vi "BMU诊断标定.vi"(5 "timeout":u32, 6 "Socket":dbl, 7 "通用配置?":bool, 8 "CAN端口":u16(ring), 9 "设备索引号":u16(ring), 10 "CAN卡类型":u32(ring)=21, 11 "从板号":u8=1) -> (3 "成功?":bool)   [LabVIEW 2013] (continued)
              tunnel: [T21."从板信息" ("等级 2") T21."从板信息" ("等级 2") T21."从板信息" ("等级 2") T21."从板信息" ("等级 2") T21."从板信息" ("等级 2") T21."从板信息" ("等级 2") T21."从板信息" ("等级 2") T21."一级故障阀值" ("等级 2") T21."二级故障阀值" ("等级 2") T21."三级故障阀值" ("等级 2") T21."快换参数" ("等级 2") T21."快换参数" ("等级 2") T21."快换参数" ("等级 2") T21."快换参数" ("等级 2") T21."快换参数" ("等级 2") T21."快换参数" ("等级 2") T21."快换参数" ("等级 2") T21."快换参数" ("等级 2") T14."均衡参数" ("等级 2") T14."均衡参数" ("等级 2") T14."均衡参数" ("等级 2") T21."从板信息" ("等级 2")] -> w2480
              tunnel: [w2493 w2503 w2517 w2532 w2567 w2604 w2641 w2665 w2678 w2691 w2704 w2730 w2744 w2760 w2777 w2794 w2812 w2831 w2848 w2861 w2875 w2890] -> w2479
              tunnel: [w2485 w2495 w2505 w2519 w2554 w2591 w2628 w2676 w2678 w2691 w2704 w2730 w2744 w2760 w2777 w2794 w2812 w2831 w2848 w2861 w2875 w2889] -> w2478
              tunnel: [w2485 w2495 w2505 w2519 w2554 w2591 w2628 w2665 w2689 w2691 w2704 w2730 w2744 w2760 w2777 w2794 w2812 w2831 w2848 w2861 w2875 w2889] -> w2477
              tunnel: [w2485 w2495 w2505 w2519 w2554 w2591 w2628 w2665 w2678 w2702 w2704 w2730 w2744 w2760 w2777 w2794 w2812 w2831 w2848 w2861 w2875 w2889] -> w2476
              tunnel: [w2485 w2495 w2505 w2519 w2554 w2591 w2628 w2665 w2678 w2691 w2728 w2742 w2758 w2775 w2792 w2810 w2829 w2846 w2848 w2861 w2875 w2889] -> w2475
              tunnel: [w2490 w2496 w2512 w2526 w2561 w2598 w2635 w2672 w2685 w2698 w2713 w2735 w2750 w2764 w2782 w2797 w2817 w2835 w2851 w2865 w2880 w2889] -> w2474
              tunnel: [w2487 w2496 w2511 w2525 w2560 w2597 w2634 w2671 w2684 w2697 w2705 w2734 w2749 w2763 w2783 w2798 w2816 w2834 w2850 w2864 w2879 w2889] -> w2473
              tunnel: w2470 -> [_ w2500 w2508 w2522 w2557 w2594 w2631 w2667 w2681 w2694 w2725 w2738 w2753 w2768 w2786 w2802 w2820 w2839 w2854 w2868 w2882 _]
              tunnel: [w2485 w2495 w2505 w2519 w2554 w2591 w2628 w2665 w2678 w2691 w2704 w2730 w2744 w2760 w2777 w2794 w2812 w2831 w2849 w2862 w2876 w2889] -> w2469
              frame "从板号" {
                w2492 = 2
                w2485 = FALSE ("1 6")
                n1778 = property on="项目信息 2" class="Tbl (严格)"("Disabled"=w2492) -> ()  [unwired: 2 in, 2 out]
                n1779 = property on="加热控制参数" class="Clust (严格)"("Disabled"=w2492) -> ()  [unwired: 2 in, 2 out]
                n1780 = property on="从板号" class="DigNum (严格)"("NumText.BGColor"=u32 6618880) -> ()  [unwired: 2 in, 2 out]
                n1781 = global read "功能码全局.vi" "16"() -> (w2489:bool[])
                n1782 = Index Array(array=w2489, index #1=4 ("索引"), index #2=6 ("索引")) -> (element #1=w2490:bool, element #2=w2487:bool)
                n1783 = Not(x=w2485) -> (.not. x?=w2493:bool)
              }
              frame "从板信息" {
                w2495 = FALSE ("1 6")
                n1784 = Select(t=0, s=w2500, f=1) -> (s? t:f=w2499:i32)
                n1785 = property on="从板号" class="DigNum (严格)"("NumText.BGColor"=u32 16777215) -> ()  [unwired: 2 in, 2 out]
                n1786 = property on="项目信息 2" class="Tbl (严格)"("Disabled"=w2499) -> ()  [unwired: 2 in, 2 out]
                n1787 = property on="加热控制参数" class="Clust (严格)"("Disabled"=w2499) -> ()  [unwired: 2 in, 2 out]
                n1788 = Not(x=w2495) -> (.not. x?=w2503:bool)
                n1789 = local read "从板项目信息"() -> (w2497:bool)
                n1790 = Not(x=w2497) -> (.not. x?=w2496:bool)
              }
              frame "风机关闭温差", "风机关闭温度", "风机开启温差", "风机开启温度", "加热关闭温差", "加热关闭温度", "加热开启温度", "加热控制参数" {
                w2505 = FALSE ("1 6")
                n1791 = property on="从板号" class="DigNum (严格)"("NumText.BGColor"=u32 16777215) -> ()  [unwired: 2 in, 2 out]
                n1792 = Select(t=0, s=w2508, f=1) -> (s? t:f=w2507:i32)
                n1793 = property on="项目信息 2" class="Tbl (严格)"("Disabled"=2) -> ()  [unwired: 2 in, 2 out]
                n1794 = property on="加热控制参数" class="Clust (严格)"("Disabled"=w2507) -> ()  [unwired: 2 in, 2 out]
                n1795 = global read "功能码全局.vi" "16"() -> (w2514:bool[])
                n1796 = Index Array(array=w2514, index #1=5 ("索引"), index #2=7 ("索引")) -> (element #1=w2512:bool, element #2=w2511:bool)
                n1797 = Not(x=w2505) -> (.not. x?=w2517:bool)
              }
              frame "电压个数" {
                w2519 = FALSE ("1 6")
                n1798 = property on="从板号" class="DigNum (严格)"("NumText.BGColor"=u32 16777215) -> ()  [unwired: 2 in, 2 out]
                n1799 = control-ref of="项目信息 2"() -> (w2530:refnum<vi>)
                n1800 = stacked-sequence {
                  tunnel: w2530 -> [w2537 w2539 w2548]
                  frame #0 {
                    n1801 = Bundle(0, 0) -> (w2536:cluster{i32, i32})  [unwired: 1 out]
                    n1802 = property class="Tbl (严格)"(reference=w2537, "Index Values"=w2536) -> ()  [unwired: 1 in, 2 out]
                  }
                  frame #1 {
                    n1803 = for {
                      N: 40 -> [_]
                      tunnel: w2539 -> [w2546]
                      i -> [w2541]
                      n1804 = Compound Arithmetic op=ADD(0 ("值"), w2541) -> (w2543:i32)
                      n1805 = Bundle(w2543, 0) -> (w2545:cluster{i32, i32})  [unwired: 1 out]
                      n1806 = property class="Tbl (严格)"(reference=w2546, "Active Cell"=w2545, "Cell BG Color"=u32 16448250) -> ()  [unwired: 1 in, 2 out]
                    }
                  }
                  frame #2 {
                    n1807 = for {
                      N: 1 -> [_]
                      tunnel: w2548 -> [w2553]
                      i -> [w2549]
                      n1808 = Bundle(w2549, 0) -> (w2552:cluster{i32, i32})  [unwired: 1 out]
                      n1809 = property class="Tbl (严格)"(reference=w2553, "Active Cell"=w2552, "Cell BG Color"=u32 6618880) -> ()  [unwired: 1 in, 2 out]
                    }
                  }
                }
                n1810 = Select(t=0, s=w2522, f=1) -> (s? t:f=w2521:i32)
                n1811 = property on="项目信息 2" class="Tbl (严格)"("Disabled"=w2521) -> ()  [unwired: 2 in, 2 out]
                n1812 = property on="加热控制参数" class="Clust (严格)"("Disabled"=2) -> ()  [unwired: 2 in, 2 out]
                n1813 = global read "功能码全局.vi" "15"() -> (w2528:bool[])
                n1814 = Index Array(array=w2528, index #1=0 ("索引"), index #2=4 ("索引")) -> (element #1=w2526:bool, element #2=w2525:bool)
                n1815 = Not(x=w2519) -> (.not. x?=w2532:bool)
              }
              frame "通道电压节数" {
                w2554 = FALSE ("1 6")
                n1816 = property on="从板号" class="DigNum (严格)"("NumText.BGColor"=u32 16777215) -> ()  [unwired: 2 in, 2 out]
                n1817 = control-ref of="项目信息 2"() -> (w2565:refnum<vi>)
                n1818 = stacked-sequence {
                  tunnel: w2565 -> [w2572 w2574 w2583]
                  frame #0 {
                    n1819 = Bundle(22, 0) -> (w2571:cluster{i32, i32})  [unwired: 1 out]
                    n1820 = property class="Tbl (严格)"(reference=w2572, "Index Values"=w2571) -> ()  [unwired: 1 in, 2 out]
                  }
                  frame #1 {
                    n1821 = for {
                      N: 40 -> [_]
                      tunnel: w2574 -> [w2581]
                      i -> [w2576]
                      n1822 = Compound Arithmetic op=ADD(0 ("值"), w2576) -> (w2578:i32)
                      n1823 = Bundle(w2578, 0) -> (w2580:cluster{i32, i32})  [unwired: 1 out]
                      n1824 = property class="Tbl (严格)"(reference=w2581, "Active Cell"=w2580, "Cell BG Color"=u32 16448250) -> ()  [unwired: 1 in, 2 out]
                    }
                  }
                  frame #2 {
                    n1825 = for {
                      N: 5 -> [_]
                      tunnel: w2583 -> [w2590]
                      i -> [w2586]
                      n1826 = Add(x=22, y=w2586) -> (x+y=w2585:i32)
                      n1827 = Bundle(w2585, 0) -> (w2589:cluster{i32, i32})  [unwired: 1 out]
                      n1828 = property class="Tbl (严格)"(reference=w2590, "Active Cell"=w2589, "Cell BG Color"=u32 6618880) -> ()  [unwired: 1 in, 2 out]
                    }
                  }
                }
                n1829 = Select(t=0, s=w2557, f=1) -> (s? t:f=w2556:i32)
                n1830 = property on="项目信息 2" class="Tbl (严格)"("Disabled"=w2556) -> ()  [unwired: 2 in, 2 out]
                n1831 = property on="加热控制参数" class="Clust (严格)"("Disabled"=2) -> ()  [unwired: 2 in, 2 out]
                n1832 = global read "功能码全局.vi" "15"() -> (w2563:bool[])
                n1833 = Index Array(array=w2563, index #1=1 ("索引"), index #2=5 ("索引")) -> (element #1=w2561:bool, element #2=w2560:bool)
                n1834 = Not(x=w2554) -> (.not. x?=w2567:bool)
              }
              frame "保险位置" {
                w2591 = FALSE ("1 6")
                n1835 = control-ref of="项目信息 2"() -> (w2602:refnum<vi>)
                n1836 = stacked-sequence {
                  tunnel: w2602 -> [w2609 w2611 w2620]
                  frame #0 {
                    n1837 = Bundle(0, 0) -> (w2608:cluster{i32, i32})  [unwired: 1 out]
                    n1838 = property class="Tbl (严格)"(reference=w2609, "Index Values"=w2608) -> ()  [unwired: 1 in, 2 out]
                  }
                  frame #1 {
                    n1839 = for {
                      N: 40 -> [_]
                      tunnel: w2611 -> [w2618]
                      i -> [w2614]
                      n1840 = Add(x=2, y=w2614) -> (x+y=w2613:i32)
                      n1841 = Bundle(w2613, 0) -> (w2617:cluster{i32, i32})  [unwired: 1 out]
                      n1842 = property class="Tbl (严格)"(reference=w2618, "Active Cell"=w2617, "Cell BG Color"=u32 16448250) -> ()  [unwired: 1 in, 2 out]
                    }
                  }
                  frame #2 {
                    n1843 = for {
                      N: 20 -> [_]
                      tunnel: w2620 -> [w2627]
                      i -> [w2623]
                      n1844 = Add(x=2, y=w2623) -> (x+y=w2622:i32)
                      n1845 = Bundle(w2622, 0) -> (w2626:cluster{i32, i32})  [unwired: 1 out]
                      n1846 = property class="Tbl (严格)"(reference=w2627, "Active Cell"=w2626, "Cell BG Color"=u32 6618880) -> ()  [unwired: 1 in, 2 out]
                    }
                  }
                }
                n1847 = property on="从板号" class="DigNum (严格)"("NumText.BGColor"=u32 16777215) -> ()  [unwired: 2 in, 2 out]
                n1848 = Select(t=0, s=w2594, f=1) -> (s? t:f=w2593:i32)
                n1849 = property on="项目信息 2" class="Tbl (严格)"("Disabled"=w2593) -> ()  [unwired: 2 in, 2 out]
                n1850 = property on="加热控制参数" class="Clust (严格)"("Disabled"=2) -> ()  [unwired: 2 in, 2 out]
                n1851 = global read "功能码全局.vi" "15"() -> (w2600:bool[])
                n1852 = Index Array(array=w2600, index #1=2 ("索引"), index #2=6 ("索引")) -> (element #1=w2598:bool, element #2=w2597:bool)
                n1853 = Not(x=w2591) -> (.not. x?=w2604:bool)
              }
              frame "温度个数" {
                w2628 = FALSE ("1 6")
                n1854 = control-ref of="项目信息 2"() -> (w2639:refnum<vi>)
                n1855 = stacked-sequence {
                  tunnel: w2639 -> [w2646 w2647 w2657]
                  frame #0 {
                    n1856 = Bundle(0, 0) -> (w2645:cluster{i32, i32})  [unwired: 1 out]
                    n1857 = property class="Tbl (严格)"(reference=w2646, "Index Values"=w2645) -> ()  [unwired: 1 in, 2 out]
                  }
                  frame #1 {
                    n1858 = for {
                      N: 40 -> [_]
                      tunnel: w2647 -> [w2655]
                      i -> [w2650]
                      n1859 = Compound Arithmetic op=ADD(0 ("值"), w2650) -> (w2652:i32)
                      n1860 = Bundle(w2652, 0) -> (w2654:cluster{i32, i32})  [unwired: 1 out]
                      n1861 = property class="Tbl (严格)"(reference=w2655, "Active Cell"=w2654, "Cell BG Color"=u32 16448250) -> ()  [unwired: 1 in, 2 out]
                    }
                  }
                  frame #2 {
                    n1862 = for {
                      N: 1 -> [_]
                      tunnel: w2657 -> [w2664]
                      i -> [w2660]
                      n1863 = Add(x=1, y=w2660) -> (x+y=w2659:i32)
                      n1864 = Bundle(w2659, 0) -> (w2663:cluster{i32, i32})  [unwired: 1 out]
                      n1865 = property class="Tbl (严格)"(reference=w2664, "Active Cell"=w2663, "Cell BG Color"=u32 6618880) -> ()  [unwired: 1 in, 2 out]
                    }
                  }
                }
                n1866 = Select(t=0, s=w2631, f=1) -> (s? t:f=w2630:i32)
                n1867 = property on="项目信息 2" class="Tbl (严格)"("Disabled"=w2630) -> ()  [unwired: 2 in, 2 out]
                n1868 = property on="加热控制参数" class="Clust (严格)"("Disabled"=2) -> ()  [unwired: 2 in, 2 out]
                n1869 = property on="从板号" class="DigNum (严格)"("NumText.BGColor"=u32 16777215) -> ()  [unwired: 2 in, 2 out]
                n1870 = global read "功能码全局.vi" "15"() -> (w2637:bool[])
                n1871 = Index Array(array=w2637, index #1=3 ("索引"), index #2=7 ("索引")) -> (element #1=w2635:bool, element #2=w2634:bool)
                n1872 = Not(x=w2628) -> (.not. x?=w2641:bool)
              }
              frame "SOC过低", "电压不均衡", "电压过低", "电压过高", "温度不均衡", "温度过低", "温度过高", "一级故障阀值" {
                w2665 = FALSE ("1 6")
                n1873 = property on="从板号" class="DigNum (严格)"("NumText.BGColor"=u32 16777215) -> ()  [unwired: 2 in, 2 out]
                n1874 = Select(t=0, s=w2667, f=1) -> (s? t:f=w2668:i32)
                n1875 = property on="一级故障 6" class="Clust (严格)"("DisabledEnum"=w2668) -> ()  [unwired: 2 in, 2 out]
                n1876 = global read "功能码全局.vi" "18"() -> (w2674:bool[])
                n1877 = Index Array(array=w2674, index #1=2 ("索引"), index #2=5 ("索引")) -> (element #1=w2672:bool, element #2=w2671:bool)
                n1878 = Not(x=w2665) -> (.not. x?=w2676:bool)
              }
              frame "SOC过低(2)", "电压不均衡(2)", "电压过低(2)", "电压过高(2)", "二级故障阀值", "温度不均衡(2)", "温度过低(2)", "温度过高(2)" {
                w2678 = FALSE ("1 6")
                n1879 = property on="从板号" class="DigNum (严格)"("NumText.BGColor"=u32 16777215) -> ()  [unwired: 2 in, 2 out]
                n1880 = Select(t=0, s=w2681, f=1) -> (s? t:f=w2680:i32)
                n1881 = property on="一级故障 7" class="Clust (严格)"("DisabledEnum"=w2680) -> ()  [unwired: 2 in, 2 out]
                n1882 = global read "功能码全局.vi" "18"() -> (w2687:bool[])
                n1883 = Index Array(array=w2687, index #1=3 ("索引"), index #2=6 ("索引")) -> (element #1=w2685:bool, element #2=w2684:bool)
                n1884 = Not(x=w2678) -> (.not. x?=w2689:bool)
              }
              frame "SOC过低(3)", "电压不均衡(3)", "电压过低(3)", "电压过高(3)", "三级故障阀值", "温度不均衡(3)", "温度过低(3)", "温度过高(3)" {
                w2691 = FALSE ("1 6")
                n1885 = property on="从板号" class="DigNum (严格)"("NumText.BGColor"=u32 16777215) -> ()  [unwired: 2 in, 2 out]
                n1886 = Select(t=0, s=w2694, f=1) -> (s? t:f=w2693:i32)
                n1887 = property on="一级故障 8" class="Clust (严格)"("DisabledEnum"=w2693) -> ()  [unwired: 2 in, 2 out]
                n1888 = global read "功能码全局.vi" "18"() -> (w2700:bool[])
                n1889 = Index Array(array=w2700, index #1=4 ("索引"), index #2=7 ("索引")) -> (element #1=w2698:bool, element #2=w2697:bool)
                n1890 = Not(x=w2691) -> (.not. x?=w2702:bool)
              }
              frame "快换参数" {
                w2704 = FALSE ("1 6")
                n1891 = Select(t=0, s=w2725, f=1) -> (s? t:f=w2724:i32)
                n1892 = property on="电池组信息" class="Clust (严格)"("Disabled"=w2724) -> ()  [unwired: 2 in, 2 out]
                n1893 = property on="从板号" class="DigNum (严格)"("NumText.BGColor"=u32 16777215) -> ()  [unwired: 2 in, 2 out]
                n1894 = global read "功能码全局.vi" "24"() -> (w2721:bool[])
                n1895 = global read "功能码全局.vi" "23"() -> (w2722:bool[])
                n1896 = Index Array(array=w2721) -> (element #3=w2711:bool, element #4=w2710:bool, element #5=w2709:bool, element #6=w2708:bool, element #7=w2707:bool, element #8=w2706:bool)  [unwired: 8 in, 2 out]
                n1897 = Index Array(array=w2722) -> (element #3=w2720:bool, element #4=w2719:bool, element #5=w2718:bool, element #6=w2717:bool, element #7=w2716:bool, element #8=w2715:bool)  [unwired: 8 in, 2 out]
                n1898 = Build Array(w2711, w2710, w2709, w2708, w2707, w2706) -> (w2712:bool[])
                n1899 = Build Array(w2720, w2719, w2718, w2717, w2716, w2715) -> (w2714:bool[])
                n1900 = And Array Elements(Boolean array=w2712) -> (logical AND=w2705:bool)
                n1901 = And Array Elements(Boolean array=w2714) -> (logical AND=w2713:bool)
                n1902 = Not(x=w2704) -> (.not. x?=w2728:bool)
              }
              frame "电池包信息1" {
                w2733 = 2
                w2741 = 2
                w2732 = 2
                w2730 = FALSE ("1 6")
                n1903 = Select(t=0, s=w2738, f=1) -> (s? t:f=w2731:i32)
                n1904 = property on="串联数" class="DigNum (严格)"("Disabled"=w2731) -> ()  [unwired: 2 in, 2 out]
                n1905 = property on="并联数" class="DigNum (严格)"("Disabled"=w2731) -> ()  [unwired: 2 in, 2 out]
                n1906 = property on="电池厂家" class="DigNum (严格)"("Disabled"=w2731) -> ()  [unwired: 2 in, 2 out]
                n1907 = property on="电池类型" class="DigNum (严格)"("Disabled"=w2731) -> ()  [unwired: 2 in, 2 out]
                n1908 = property on="额定能量" class="DigNum (严格)"("Disabled"=w2731) -> ()  [unwired: 2 in, 2 out]
                n1909 = property on="额定容量" class="DigNum (严格)"("Disabled"=w2731) -> ()  [unwired: 2 in, 2 out]
                n1910 = property on="实际容量" class="DigNum (严格)"("Disabled"=w2731) -> ()  [unwired: 2 in, 2 out]
                n1911 = property on="电池组信息" class="Clust (严格)"("Disabled"=w2731) -> ()  [unwired: 2 in, 2 out]
                n1912 = property on="生产日期" class="Str"("DisabledEnum"=w2731) -> ()  [unwired: 2 in, 2 out]
                n1913 = property on="车牌号" class="Str"("DisabledEnum"=w2732) -> ()  [unwired: 2 in, 2 out]
                n1914 = property on="产权标识" class="DigNum (严格)"("Disabled"=w2731) -> ()  [unwired: 2 in, 2 out]
                n1915 = property on="应用车型" class="DigNum (严格)"("Disabled"=w2731) -> ()  [unwired: 2 in, 2 out]
                n1916 = property on="额定总压" class="DigNum (严格)"("Disabled"=w2731) -> ()  [unwired: 2 in, 2 out]
                n1917 = property on="电池包序号" class="DigNum (严格)"("DisabledEnum"=w2731) -> ()  [unwired: 2 in, 2 out]
                n1918 = property on="电池包组号" class="DigNum (严格)"("DisabledEnum"=w2732) -> ()  [unwired: 2 in, 2 out]
                n1919 = property on="最大允许单体电压" class="DigNum (严格)"("Disabled"=w2741) -> ()  [unwired: 2 in, 2 out]
                n1920 = property on="最大允许总电压" class="DigNum (严格)"("Disabled"=w2741) -> ()  [unwired: 2 in, 2 out]
                n1921 = property on="最大允许温度" class="DigNum (严格)"("Disabled"=w2741) -> ()  [unwired: 2 in, 2 out]
                n1922 = property on="最小允许温度" class="DigNum (严格)"("Disabled"=w2741) -> ()  [unwired: 2 in, 2 out]
                n1923 = property on="最大允许充电电流" class="DigNum (严格)"("Disabled"=w2741) -> ()  [unwired: 2 in, 2 out]
                n1924 = property on="最小允许充电电流" class="DigNum (严格)"("Disabled"=w2741) -> ()  [unwired: 2 in, 2 out]
                n1925 = property on="最小允许单体电压" class="DigNum (严格)"("Disabled"=w2741) -> ()  [unwired: 2 in, 2 out]
                n1926 = property on="电流步长" class="DigNum (严格)"("Disabled"=w2741) -> ()  [unwired: 2 in, 2 out]
                n1927 = property on="SOC" class="DigNum (严格)"("Disabled"=w2741) -> ()  [unwired: 2 in, 2 out]
                n1928 = property on="充电总安时" class="DigNum (严格)"("Disabled"=w2741) -> ()  [unwired: 2 in, 2 out]
                n1929 = property on="放电总安时" class="DigNum (严格)"("Disabled"=w2741) -> ()  [unwired: 2 in, 2 out]
                n1930 = property on="放空次数" class="DigNum (严格)"("DisabledEnum"=w2733) -> ()  [unwired: 2 in, 2 out]
                n1931 = property on="充满次数" class="DigNum (严格)"("DisabledEnum"=w2733) -> ()  [unwired: 2 in, 2 out]
                n1932 = property on="充电次数" class="DigNum (严格)"("DisabledEnum"=w2733) -> ()  [unwired: 2 in, 2 out]
                n1933 = global read "功能码全局.vi" "24"() -> (w2736:bool[])
                n1934 = global read "功能码全局.vi" "23"() -> (w2737:bool[])
                n1935 = Index Array(array=w2736) -> (element #3=w2734:bool)  [unwired: 8 in, 7 out]
                n1936 = Index Array(array=w2737) -> (element #3=w2735:bool)  [unwired: 8 in, 7 out]
                n1937 = Not(x=w2730) -> (.not. x?=w2742:bool)
              }
              frame "电池包组号" {
                w2747 = 2
                w2746 = 2
                w2756 = 2
                w2748 = 2
                w2757 = 2
                w2744 = FALSE ("1 6")
                n1938 = property on="串联数" class="DigNum (严格)"("Disabled"=w2757) -> ()  [unwired: 2 in, 2 out]
                n1939 = property on="并联数" class="DigNum (严格)"("Disabled"=w2757) -> ()  [unwired: 2 in, 2 out]
                n1940 = property on="电池厂家" class="DigNum (严格)"("Disabled"=w2757) -> ()  [unwired: 2 in, 2 out]
                n1941 = property on="电池类型" class="DigNum (严格)"("Disabled"=w2757) -> ()  [unwired: 2 in, 2 out]
                n1942 = property on="额定能量" class="DigNum (严格)"("Disabled"=w2757) -> ()  [unwired: 2 in, 2 out]
                n1943 = property on="额定容量" class="DigNum (严格)"("Disabled"=w2757) -> ()  [unwired: 2 in, 2 out]
                n1944 = property on="实际容量" class="DigNum (严格)"("Disabled"=w2757) -> ()  [unwired: 2 in, 2 out]
                n1945 = Select(t=0, s=w2753, f=1) -> (s? t:f=w2745:i32)
                n1946 = property on="生产日期" class="Str"("DisabledEnum"=w2747) -> ()  [unwired: 2 in, 2 out]
                n1947 = property on="电池包序号" class="DigNum (严格)"("DisabledEnum"=w2747) -> ()  [unwired: 2 in, 2 out]
                n1948 = property on="车牌号" class="Str"("DisabledEnum"=w2747) -> ()  [unwired: 2 in, 2 out]
                n1949 = property on="电池包组号" class="DigNum (严格)"("DisabledEnum"=w2745) -> ()  [unwired: 2 in, 2 out]
                n1950 = property on="电池组信息" class="Clust (严格)"("Disabled"=w2745) -> ()  [unwired: 2 in, 2 out]
                n1951 = property on="产权标识" class="DigNum (严格)"("Disabled"=w2748) -> ()  [unwired: 2 in, 2 out]
                n1952 = property on="应用车型" class="DigNum (严格)"("Disabled"=w2748) -> ()  [unwired: 2 in, 2 out]
                n1953 = property on="额定总压" class="DigNum (严格)"("Disabled"=w2748) -> ()  [unwired: 2 in, 2 out]
                n1954 = property on="放空次数" class="DigNum (严格)"("DisabledEnum"=w2746) -> ()  [unwired: 2 in, 2 out]
                n1955 = property on="充满次数" class="DigNum (严格)"("DisabledEnum"=w2746) -> ()  [unwired: 2 in, 2 out]
                n1956 = property on="充电次数" class="DigNum (严格)"("DisabledEnum"=w2746) -> ()  [unwired: 2 in, 2 out]
                n1957 = property on="最大允许单体电压" class="DigNum (严格)"("Disabled"=w2756) -> ()  [unwired: 2 in, 2 out]
                n1958 = property on="最大允许总电压" class="DigNum (严格)"("Disabled"=w2756) -> ()  [unwired: 2 in, 2 out]
                n1959 = property on="最大允许温度" class="DigNum (严格)"("Disabled"=w2756) -> ()  [unwired: 2 in, 2 out]
                n1960 = property on="最小允许温度" class="DigNum (严格)"("Disabled"=w2756) -> ()  [unwired: 2 in, 2 out]
                n1961 = property on="最大允许充电电流" class="DigNum (严格)"("Disabled"=w2756) -> ()  [unwired: 2 in, 2 out]
                n1962 = property on="最小允许充电电流" class="DigNum (严格)"("Disabled"=w2756) -> ()  [unwired: 2 in, 2 out]
                n1963 = property on="最小允许单体电压" class="DigNum (严格)"("Disabled"=w2756) -> ()  [unwired: 2 in, 2 out]
                n1964 = property on="电流步长" class="DigNum (严格)"("Disabled"=w2756) -> ()  [unwired: 2 in, 2 out]
                n1965 = property on="SOC" class="DigNum (严格)"("Disabled"=w2756) -> ()  [unwired: 2 in, 2 out]
                n1966 = property on="充电总安时" class="DigNum (严格)"("Disabled"=w2756) -> ()  [unwired: 2 in, 2 out]
                n1967 = property on="放电总安时" class="DigNum (严格)"("Disabled"=w2756) -> ()  [unwired: 2 in, 2 out]
                n1968 = global read "功能码全局.vi" "24"() -> (w2751:bool[])
                n1969 = global read "功能码全局.vi" "23"() -> (w2752:bool[])
                n1970 = Index Array(array=w2751) -> (element #3=w2749:bool)  [unwired: 8 in, 7 out]
                n1971 = Index Array(array=w2752) -> (element #3=w2750:bool)  [unwired: 8 in, 7 out]
                n1972 = Not(x=w2744) -> (.not. x?=w2758:bool)
              }
              frame "充放电安时" {
                w2762 = 2
                w2761 = 2
                w2771 = 2
                w2772 = 2
                w2774 = 2
                w2760 = FALSE ("1 6")
                n1973 = property on="串联数" class="DigNum (严格)"("Disabled"=w2774) -> ()  [unwired: 2 in, 2 out]
                n1974 = property on="并联数" class="DigNum (严格)"("Disabled"=w2774) -> ()  [unwired: 2 in, 2 out]
                n1975 = property on="电池厂家" class="DigNum (严格)"("Disabled"=w2774) -> ()  [unwired: 2 in, 2 out]
                n1976 = property on="电池类型" class="DigNum (严格)"("Disabled"=w2774) -> ()  [unwired: 2 in, 2 out]
                n1977 = property on="额定能量" class="DigNum (严格)"("Disabled"=w2774) -> ()  [unwired: 2 in, 2 out]
                n1978 = property on="额定容量" class="DigNum (严格)"("Disabled"=w2774) -> ()  [unwired: 2 in, 2 out]
                n1979 = property on="实际容量" class="DigNum (严格)"("Disabled"=w2774) -> ()  [unwired: 2 in, 2 out]
                n1980 = Select(t=0, s=w2768, f=1) -> (s? t:f=w2767:i32)
                n1981 = property on="生产日期" class="Str"("DisabledEnum"=w2762) -> ()  [unwired: 2 in, 2 out]
                n1982 = property on="电池包序号" class="DigNum (严格)"("DisabledEnum"=w2762) -> ()  [unwired: 2 in, 2 out]
                n1983 = property on="车牌号" class="Str"("DisabledEnum"=w2762) -> ()  [unwired: 2 in, 2 out]
                n1984 = property on="电池包组号" class="DigNum (严格)"("DisabledEnum"=w2762) -> ()  [unwired: 2 in, 2 out]
                n1985 = property on="电池组信息" class="Clust (严格)"("Disabled"=w2767) -> ()  [unwired: 2 in, 2 out]
                n1986 = property on="额定总压" class="DigNum (严格)"("Disabled"=2) -> ()  [unwired: 2 in, 2 out]
                n1987 = property on="产权标识" class="DigNum (严格)"("Disabled"=w2772) -> ()  [unwired: 2 in, 2 out]
                n1988 = property on="应用车型" class="DigNum (严格)"("Disabled"=w2772) -> ()  [unwired: 2 in, 2 out]
                n1989 = property on="放空次数" class="DigNum (严格)"("DisabledEnum"=w2761) -> ()  [unwired: 2 in, 2 out]
                n1990 = property on="充满次数" class="DigNum (严格)"("DisabledEnum"=w2761) -> ()  [unwired: 2 in, 2 out]
                n1991 = property on="充电次数" class="DigNum (严格)"("DisabledEnum"=w2761) -> ()  [unwired: 2 in, 2 out]
                n1992 = property on="最大允许单体电压" class="DigNum (严格)"("Disabled"=w2771) -> ()  [unwired: 2 in, 2 out]
                n1993 = property on="最大允许总电压" class="DigNum (严格)"("Disabled"=w2771) -> ()  [unwired: 2 in, 2 out]
                n1994 = property on="最大允许温度" class="DigNum (严格)"("Disabled"=w2771) -> ()  [unwired: 2 in, 2 out]
                n1995 = property on="最小允许温度" class="DigNum (严格)"("Disabled"=w2771) -> ()  [unwired: 2 in, 2 out]
                n1996 = property on="最大允许充电电流" class="DigNum (严格)"("Disabled"=w2771) -> ()  [unwired: 2 in, 2 out]
                n1997 = property on="最小允许充电电流" class="DigNum (严格)"("Disabled"=w2771) -> ()  [unwired: 2 in, 2 out]
                n1998 = property on="最小允许单体电压" class="DigNum (严格)"("Disabled"=w2771) -> ()  [unwired: 2 in, 2 out]
                n1999 = property on="电流步长" class="DigNum (严格)"("Disabled"=w2771) -> ()  [unwired: 2 in, 2 out]
                n2000 = property on="SOC" class="DigNum (严格)"("Disabled"=w2771) -> ()  [unwired: 2 in, 2 out]
                n2001 = property on="充电总安时" class="DigNum (严格)"("Disabled"=w2767) -> ()  [unwired: 2 in, 2 out]
                n2002 = property on="放电总安时" class="DigNum (严格)"("Disabled"=w2767) -> ()  [unwired: 2 in, 2 out]
                n2003 = Not(x=w2760) -> (.not. x?=w2775:bool)
                n2004 = global read "功能码全局.vi" "24"() -> (w2765:bool[])
                n2005 = global read "功能码全局.vi" "23"() -> (w2766:bool[])
                n2006 = Index Array(array=w2765) -> (element #7=w2763:bool)  [unwired: 8 in, 7 out]
                n2007 = Index Array(array=w2766) -> (element #7=w2764:bool)  [unwired: 8 in, 7 out]
              }
              frame "充电次数" {
                w2780 = 2
                w2789 = 2
                w2790 = 2
                w2781 = 2
                w2791 = 2
                w2777 = FALSE ("1 6")
                n2008 = property on="串联数" class="DigNum (严格)"("Disabled"=w2791) -> ()  [unwired: 2 in, 2 out]
                n2009 = property on="并联数" class="DigNum (严格)"("Disabled"=w2791) -> ()  [unwired: 2 in, 2 out]
                n2010 = property on="电池厂家" class="DigNum (严格)"("Disabled"=w2791) -> ()  [unwired: 2 in, 2 out]
                n2011 = property on="电池类型" class="DigNum (严格)"("Disabled"=w2791) -> ()  [unwired: 2 in, 2 out]
                n2012 = property on="额定能量" class="DigNum (严格)"("Disabled"=w2791) -> ()  [unwired: 2 in, 2 out]
                n2013 = property on="额定容量" class="DigNum (严格)"("Disabled"=w2791) -> ()  [unwired: 2 in, 2 out]
                n2014 = property on="实际容量" class="DigNum (严格)"("Disabled"=w2791) -> ()  [unwired: 2 in, 2 out]
                n2015 = Select(t=0, s=w2786, f=1) -> (s? t:f=w2778:i32)
                n2016 = property on="生产日期" class="Str"("DisabledEnum"=w2780) -> ()  [unwired: 2 in, 2 out]
                n2017 = property on="电池包序号" class="DigNum (严格)"("DisabledEnum"=w2780) -> ()  [unwired: 2 in, 2 out]
                n2018 = property on="车牌号" class="Str"("DisabledEnum"=w2780) -> ()  [unwired: 2 in, 2 out]
                n2019 = property on="电池组信息" class="Clust (严格)"("Disabled"=w2778) -> ()  [unwired: 2 in, 2 out]
                n2020 = property on="电池包组号" class="DigNum (严格)"("DisabledEnum"=w2780) -> ()  [unwired: 2 in, 2 out]
                n2021 = property on="额定总压" class="DigNum (严格)"("Disabled"=w2781) -> ()  [unwired: 2 in, 2 out]
                n2022 = property on="产权标识" class="DigNum (严格)"("Disabled"=w2781) -> ()  [unwired: 2 in, 2 out]
                n2023 = property on="应用车型" class="DigNum (严格)"("Disabled"=w2781) -> ()  [unwired: 2 in, 2 out]
                n2024 = property on="放空次数" class="DigNum (严格)"("DisabledEnum"=w2778) -> (error out=w2779:errorcluster)  [unwired: 2 in, 1 out]
                n2025 = property on="充满次数" class="DigNum (严格)"("DisabledEnum"=w2778) -> ()  [unwired: 2 in, 2 out]
                n2026 = property on="充电次数" class="DigNum (严格)"("DisabledEnum"=w2778) -> ()  [unwired: 2 in, 2 out]
                n2027 = property on="最大允许单体电压" class="DigNum (严格)"("Disabled"=w2790) -> ()  [unwired: 2 in, 2 out]
                n2028 = property on="最大允许总电压" class="DigNum (严格)"("Disabled"=w2790) -> ()  [unwired: 2 in, 2 out]
                n2029 = property on="最大允许温度" class="DigNum (严格)"("Disabled"=w2790) -> ()  [unwired: 2 in, 2 out]
                n2030 = property on="最小允许温度" class="DigNum (严格)"("Disabled"=w2790) -> ()  [unwired: 2 in, 2 out]
                n2031 = property on="最大允许充电电流" class="DigNum (严格)"("Disabled"=w2790) -> ()  [unwired: 2 in, 2 out]
                n2032 = property on="最小允许充电电流" class="DigNum (严格)"(error in=w2779, "Disabled"=w2790) -> ()  [unwired: 1 in, 2 out]
                n2033 = property on="最小允许单体电压" class="DigNum (严格)"("Disabled"=w2790) -> ()  [unwired: 2 in, 2 out]
                n2034 = property on="电流步长" class="DigNum (严格)"("Disabled"=w2790) -> ()  [unwired: 2 in, 2 out]
                n2035 = property on="SOC" class="DigNum (严格)"("Disabled"=w2790) -> ()  [unwired: 2 in, 2 out]
                n2036 = property on="充电总安时" class="DigNum (严格)"("Disabled"=w2789) -> ()  [unwired: 2 in, 2 out]
                n2037 = property on="放电总安时" class="DigNum (严格)"("Disabled"=w2789) -> ()  [unwired: 2 in, 2 out]
                n2038 = Not(x=w2777) -> (.not. x?=w2792:bool)
                n2039 = global read "功能码全局.vi" "24"() -> (w2784:bool[])
                n2040 = global read "功能码全局.vi" "23"() -> (w2785:bool[])
                n2041 = Index Array(array=w2784) -> (element #8=w2783:bool)  [unwired: 8 in, 7 out]
                n2042 = Index Array(array=w2785) -> (element #8=w2782:bool)  [unwired: 8 in, 7 out]
              }
              frame "SOC" {
                w2796 = 2
                w2795 = 2
                w2805 = 2
                w2806 = 2
                w2807 = 2
                w2809 = 2
                w2794 = FALSE ("1 6")
                n2043 = property on="串联数" class="DigNum (严格)"("Disabled"=w2809) -> ()  [unwired: 2 in, 2 out]
                n2044 = property on="并联数" class="DigNum (严格)"("Disabled"=w2809) -> ()  [unwired: 2 in, 2 out]
                n2045 = property on="电池厂家" class="DigNum (严格)"("Disabled"=w2809) -> ()  [unwired: 2 in, 2 out]
                n2046 = property on="电池类型" class="DigNum (严格)"("Disabled"=w2809) -> ()  [unwired: 2 in, 2 out]
                n2047 = property on="额定能量" class="DigNum (严格)"("Disabled"=w2809) -> ()  [unwired: 2 in, 2 out]
                n2048 = property on="额定容量" class="DigNum (严格)"("Disabled"=w2809) -> ()  [unwired: 2 in, 2 out]
                n2049 = property on="实际容量" class="DigNum (严格)"("Disabled"=w2809) -> ()  [unwired: 2 in, 2 out]
                n2050 = Select(t=0, s=w2802, f=1) -> (s? t:f=w2801:i32)
                n2051 = property on="生产日期" class="Str"("DisabledEnum"=w2796) -> ()  [unwired: 2 in, 2 out]
                n2052 = property on="电池包序号" class="DigNum (严格)"("DisabledEnum"=w2796) -> ()  [unwired: 2 in, 2 out]
                n2053 = property on="车牌号" class="Str"("DisabledEnum"=w2796) -> ()  [unwired: 2 in, 2 out]
                n2054 = property on="电池包组号" class="DigNum (严格)"("DisabledEnum"=w2796) -> ()  [unwired: 2 in, 2 out]
                n2055 = property on="电池组信息" class="Clust (严格)"("Disabled"=w2801) -> ()  [unwired: 2 in, 2 out]
                n2056 = property on="SOC" class="DigNum (严格)"("Disabled"=w2801) -> ()  [unwired: 2 in, 2 out]
                n2057 = property on="额定总压" class="DigNum (严格)"("Disabled"=2) -> ()  [unwired: 2 in, 2 out]
                n2058 = property on="产权标识" class="DigNum (严格)"("Disabled"=w2807) -> ()  [unwired: 2 in, 2 out]
                n2059 = property on="应用车型" class="DigNum (严格)"("Disabled"=w2807) -> ()  [unwired: 2 in, 2 out]
                n2060 = property on="放空次数" class="DigNum (严格)"("DisabledEnum"=w2795) -> ()  [unwired: 2 in, 2 out]
                n2061 = property on="充满次数" class="DigNum (严格)"("DisabledEnum"=w2795) -> ()  [unwired: 2 in, 2 out]
                n2062 = property on="充电次数" class="DigNum (严格)"("DisabledEnum"=w2795) -> ()  [unwired: 2 in, 2 out]
                n2063 = property on="最大允许单体电压" class="DigNum (严格)"("Disabled"=w2806) -> ()  [unwired: 2 in, 2 out]
                n2064 = property on="最大允许总电压" class="DigNum (严格)"("Disabled"=w2806) -> ()  [unwired: 2 in, 2 out]
                n2065 = property on="最大允许温度" class="DigNum (严格)"("Disabled"=w2806) -> ()  [unwired: 2 in, 2 out]
                n2066 = property on="最小允许温度" class="DigNum (严格)"("Disabled"=w2806) -> ()  [unwired: 2 in, 2 out]
                n2067 = property on="最大允许充电电流" class="DigNum (严格)"("Disabled"=w2806) -> ()  [unwired: 2 in, 2 out]
                n2068 = property on="最小允许充电电流" class="DigNum (严格)"("Disabled"=w2806) -> ()  [unwired: 2 in, 2 out]
                n2069 = property on="最小允许单体电压" class="DigNum (严格)"("Disabled"=w2806) -> ()  [unwired: 2 in, 2 out]
                n2070 = property on="电流步长" class="DigNum (严格)"("Disabled"=w2806) -> ()  [unwired: 2 in, 2 out]
                n2071 = property on="充电总安时" class="DigNum (严格)"("Disabled"=w2805) -> ()  [unwired: 2 in, 2 out]
                n2072 = property on="放电总安时" class="DigNum (严格)"("Disabled"=w2805) -> ()  [unwired: 2 in, 2 out]
                n2073 = Not(x=w2794) -> (.not. x?=w2810:bool)
                n2074 = global read "功能码全局.vi" "24"() -> (w2799:bool[])
                n2075 = global read "功能码全局.vi" "23"() -> (w2800:bool[])
                n2076 = Index Array(array=w2799) -> (element #6=w2798:bool)  [unwired: 8 in, 7 out]
                n2077 = Index Array(array=w2800) -> (element #6=w2797:bool)  [unwired: 8 in, 7 out]
              }
              frame "车牌号" {
                w2815 = 2
                w2814 = 2
                w2824 = 2
                w2825 = 2
                w2826 = 2
                w2828 = 2
                w2812 = FALSE ("1 6")
                n2078 = property on="串联数" class="DigNum (严格)"("Disabled"=w2828) -> ()  [unwired: 2 in, 2 out]
                n2079 = property on="并联数" class="DigNum (严格)"("Disabled"=w2828) -> ()  [unwired: 2 in, 2 out]
                n2080 = property on="电池厂家" class="DigNum (严格)"("Disabled"=w2828) -> ()  [unwired: 2 in, 2 out]
                n2081 = property on="电池类型" class="DigNum (严格)"("Disabled"=w2828) -> ()  [unwired: 2 in, 2 out]
                n2082 = property on="额定能量" class="DigNum (严格)"("Disabled"=w2828) -> ()  [unwired: 2 in, 2 out]
                n2083 = property on="额定容量" class="DigNum (严格)"("Disabled"=w2828) -> ()  [unwired: 2 in, 2 out]
                n2084 = property on="实际容量" class="DigNum (严格)"("Disabled"=w2828) -> ()  [unwired: 2 in, 2 out]
                n2085 = Select(t=0, s=w2820, f=1) -> (s? t:f=w2813:i32)
                n2086 = property on="生产日期" class="Str"("DisabledEnum"=w2815) -> ()  [unwired: 2 in, 2 out]
                n2087 = property on="电池包序号" class="DigNum (严格)"("DisabledEnum"=w2815) -> ()  [unwired: 2 in, 2 out]
                n2088 = property on="电池包组号" class="DigNum (严格)"("DisabledEnum"=w2815) -> ()  [unwired: 2 in, 2 out]
                n2089 = property on="电池组信息" class="Clust (严格)"("Disabled"=w2813) -> ()  [unwired: 2 in, 2 out]
                n2090 = property on="车牌号" class="Str"("DisabledEnum"=w2813) -> ()  [unwired: 2 in, 2 out]
                n2091 = property on="额定总压" class="DigNum (严格)"("Disabled"=2) -> ()  [unwired: 2 in, 2 out]
                n2092 = property on="产权标识" class="DigNum (严格)"("Disabled"=w2826) -> ()  [unwired: 2 in, 2 out]
                n2093 = property on="应用车型" class="DigNum (严格)"("Disabled"=w2826) -> ()  [unwired: 2 in, 2 out]
                n2094 = property on="放空次数" class="DigNum (严格)"("DisabledEnum"=w2814) -> ()  [unwired: 2 in, 2 out]
                n2095 = property on="充满次数" class="DigNum (严格)"("DisabledEnum"=w2814) -> ()  [unwired: 2 in, 2 out]
                n2096 = property on="充电次数" class="DigNum (严格)"("DisabledEnum"=w2814) -> ()  [unwired: 2 in, 2 out]
                n2097 = property on="最大允许单体电压" class="DigNum (严格)"("Disabled"=w2825) -> ()  [unwired: 2 in, 2 out]
                n2098 = property on="最大允许总电压" class="DigNum (严格)"("Disabled"=w2825) -> ()  [unwired: 2 in, 2 out]
                n2099 = property on="最大允许温度" class="DigNum (严格)"("Disabled"=w2825) -> ()  [unwired: 2 in, 2 out]
                n2100 = property on="最小允许温度" class="DigNum (严格)"("Disabled"=w2825) -> ()  [unwired: 2 in, 2 out]
                n2101 = property on="最大允许充电电流" class="DigNum (严格)"("Disabled"=w2825) -> ()  [unwired: 2 in, 2 out]
                n2102 = property on="最小允许充电电流" class="DigNum (严格)"("Disabled"=w2825) -> ()  [unwired: 2 in, 2 out]
                n2103 = property on="最小允许单体电压" class="DigNum (严格)"("Disabled"=w2825) -> ()  [unwired: 2 in, 2 out]
                n2104 = property on="电流步长" class="DigNum (严格)"("Disabled"=w2825) -> ()  [unwired: 2 in, 2 out]
                n2105 = property on="SOC" class="DigNum (严格)"("Disabled"=2) -> ()  [unwired: 2 in, 2 out]
                n2106 = property on="充电总安时" class="DigNum (严格)"("Disabled"=w2824) -> ()  [unwired: 2 in, 2 out]
                n2107 = property on="放电总安时" class="DigNum (严格)"("Disabled"=w2824) -> ()  [unwired: 2 in, 2 out]
                n2108 = Not(x=w2812) -> (.not. x?=w2829:bool)
                n2109 = global read "功能码全局.vi" "24"() -> (w2818:bool[])
                n2110 = global read "功能码全局.vi" "23"() -> (w2819:bool[])
                n2111 = Index Array(array=w2818) -> (element #5=w2816:bool)  [unwired: 8 in, 7 out]
                n2112 = Index Array(array=w2819) -> (element #5=w2817:bool)  [unwired: 8 in, 7 out]
              }
              frame "充电参数" {
                w2833 = 2
                w2832 = 2
                w2842 = 2
                w2843 = 2
                w2845 = 2
                w2831 = FALSE ("1 6")
                n2113 = property on="串联数" class="DigNum (严格)"("Disabled"=w2845) -> ()  [unwired: 2 in, 2 out]
                n2114 = property on="并联数" class="DigNum (严格)"("Disabled"=w2845) -> ()  [unwired: 2 in, 2 out]
                n2115 = property on="电池厂家" class="DigNum (严格)"("Disabled"=w2845) -> ()  [unwired: 2 in, 2 out]
                n2116 = property on="电池类型" class="DigNum (严格)"("Disabled"=w2845) -> ()  [unwired: 2 in, 2 out]
                n2117 = property on="额定能量" class="DigNum (严格)"("Disabled"=w2845) -> ()  [unwired: 2 in, 2 out]
                n2118 = property on="额定容量" class="DigNum (严格)"("Disabled"=w2845) -> ()  [unwired: 2 in, 2 out]
                n2119 = property on="实际容量" class="DigNum (严格)"("Disabled"=w2845) -> ()  [unwired: 2 in, 2 out]
                n2120 = Select(t=0, s=w2839, f=1) -> (s? t:f=w2838:i32)
                n2121 = property on="生产日期" class="Str"("DisabledEnum"=w2833) -> ()  [unwired: 2 in, 2 out]
                n2122 = property on="电池包序号" class="DigNum (严格)"("DisabledEnum"=w2833) -> ()  [unwired: 2 in, 2 out]
                n2123 = property on="车牌号" class="Str"("DisabledEnum"=w2833) -> ()  [unwired: 2 in, 2 out]
                n2124 = property on="电池组信息" class="Clust (严格)"("Disabled"=w2838) -> ()  [unwired: 2 in, 2 out]
                n2125 = property on="电池包组号" class="DigNum (严格)"("DisabledEnum"=w2833) -> ()  [unwired: 2 in, 2 out]
                n2126 = property on="额定总压" class="DigNum (严格)"("Disabled"=2) -> ()  [unwired: 2 in, 2 out]
                n2127 = property on="产权标识" class="DigNum (严格)"("Disabled"=w2843) -> ()  [unwired: 2 in, 2 out]
                n2128 = property on="应用车型" class="DigNum (严格)"("Disabled"=w2843) -> ()  [unwired: 2 in, 2 out]
                n2129 = property on="放空次数" class="DigNum (严格)"("DisabledEnum"=w2832) -> ()  [unwired: 2 in, 2 out]
                n2130 = property on="充满次数" class="DigNum (严格)"("DisabledEnum"=w2832) -> ()  [unwired: 2 in, 2 out]
                n2131 = property on="充电次数" class="DigNum (严格)"("DisabledEnum"=w2832) -> ()  [unwired: 2 in, 2 out]
                n2132 = property on="最大允许单体电压" class="DigNum (严格)"("Disabled"=w2838) -> ()  [unwired: 2 in, 2 out]
                n2133 = property on="最大允许总电压" class="DigNum (严格)"("Disabled"=w2838) -> ()  [unwired: 2 in, 2 out]
                n2134 = property on="最大允许温度" class="DigNum (严格)"("Disabled"=w2838) -> ()  [unwired: 2 in, 2 out]
                n2135 = property on="最小允许温度" class="DigNum (严格)"("Disabled"=w2838) -> ()  [unwired: 2 in, 2 out]
                n2136 = property on="最大允许充电电流" class="DigNum (严格)"("Disabled"=w2838) -> ()  [unwired: 2 in, 2 out]
                n2137 = property on="最小允许充电电流" class="DigNum (严格)"("Disabled"=w2838) -> ()  [unwired: 2 in, 2 out]
                n2138 = property on="最小允许单体电压" class="DigNum (严格)"("Disabled"=w2838) -> ()  [unwired: 2 in, 2 out]
                n2139 = property on="电流步长" class="DigNum (严格)"("Disabled"=w2838) -> ()  [unwired: 2 in, 2 out]
                n2140 = property on="SOC" class="DigNum (严格)"("Disabled"=w2842) -> ()  [unwired: 2 in, 2 out]
                n2141 = property on="充电总安时" class="DigNum (严格)"("Disabled"=w2842) -> ()  [unwired: 2 in, 2 out]
                n2142 = property on="放电总安时" class="DigNum (严格)"("Disabled"=w2842) -> ()  [unwired: 2 in, 2 out]
                n2143 = Not(x=w2831) -> (.not. x?=w2846:bool)
                n2144 = global read "功能码全局.vi" "24"() -> (w2836:bool[])
                n2145 = global read "功能码全局.vi" "23"() -> (w2837:bool[])
                n2146 = Index Array(array=w2836) -> (element #4=w2834:bool)  [unwired: 8 in, 7 out]
                n2147 = Index Array(array=w2837) -> (element #4=w2835:bool)  [unwired: 8 in, 7 out]
              }
              frame "均衡参数" {
                w2848 = FALSE ("1 6")
                n2148 = Select(t=0, s=w2854, f=1) -> (s? t:f=w2852:i32)
                n2149 = property on="均衡计算-电压高阀值1级" class="DigNum (严格)"("DisabledEnum"=w2852) -> ()  [unwired: 2 in, 2 out]
                n2150 = property on="均衡计算-电压高阀值2级" class="DigNum (严格)"("DisabledEnum"=w2852) -> ()  [unwired: 2 in, 2 out]
                n2151 = property on="均衡计算-电压低阀值1级" class="DigNum (严格)"("DisabledEnum"=w2852) -> ()  [unwired: 2 in, 2 out]
                n2152 = property on="均衡计算-电压低阀值2级" class="DigNum (严格)"("DisabledEnum"=w2852) -> ()  [unwired: 2 in, 2 out]
                n2153 = property on="均衡计算-最低电压阀值" class="DigNum (严格)"("DisabledEnum"=w2852) -> ()  [unwired: 2 in, 2 out]
                n2154 = property on="均衡停止-最低电压阀值" class="DigNum (严格)"("DisabledEnum"=w2852) -> ()  [unwired: 2 in, 2 out]
                n2155 = property on="均衡计算-电压极差阀值" class="DigNum (严格)"("DisabledEnum"=w2852) -> ()  [unwired: 2 in, 2 out]
                n2156 = property on="均衡参数" class="Clust (严格)"("DisabledEnum"=w2852) -> ()  [unwired: 2 in, 2 out]
                n2157 = property on="充电结束电压(90%)" class="DigNum (严格)"("DisabledEnum"=w2852) -> ()  [unwired: 2 in, 2 out]
                n2158 = property on="充电结束电压(91%)" class="DigNum (严格)"("DisabledEnum"=w2852) -> ()  [unwired: 2 in, 2 out]
                n2159 = property on="充电结束电压(92%)" class="DigNum (严格)"("DisabledEnum"=w2852) -> ()  [unwired: 2 in, 2 out]
                n2160 = property on="充电结束电压(93%)" class="DigNum (严格)"("DisabledEnum"=w2852) -> ()  [unwired: 2 in, 2 out]
                n2161 = property on="充电结束电压(94%)" class="DigNum (严格)"("DisabledEnum"=w2852) -> ()  [unwired: 2 in, 2 out]
                n2162 = property on="充电结束电压(95%)" class="DigNum (严格)"("DisabledEnum"=w2852) -> ()  [unwired: 2 in, 2 out]
                n2163 = property on="充电结束电压(96%)" class="DigNum (严格)"("DisabledEnum"=w2852) -> ()  [unwired: 2 in, 2 out]
                n2164 = property on="充电结束电压(97%)" class="DigNum (严格)"("DisabledEnum"=w2852) -> ()  [unwired: 2 in, 2 out]
                n2165 = property on="充电结束电压(98%)" class="DigNum (严格)"("DisabledEnum"=w2852) -> ()  [unwired: 2 in, 2 out]
                n2166 = property on="充电结束电压(99%)" class="DigNum (严格)"("DisabledEnum"=w2852) -> ()  [unwired: 2 in, 2 out]
                n2167 = property on="充电结束电压(100%)" class="DigNum (严格)"("DisabledEnum"=w2852) -> ()  [unwired: 2 in, 2 out]
                n2168 = disable-structure shown="启用" {
                  disable-tunnel: [w2858 w2860] -> w2851
                  disable-tunnel: [w2857 w2860] -> w2850
                  frame Enabled {
                    n2169 = global read "功能码全局.vi" "18"() -> (w2859:bool[])
                    n2170 = Index Array(array=w2859) -> (element #1=w2858:bool, element #2=w2857:bool)  [unwired: 8 in, 6 out]
                  }
                  frame Disabled {
                    w2860 = TRUE
                  }
                }
                n2171 = Not(x=w2848) -> (.not. x?=w2849:bool)
              }
              frame "均衡阀值" {
                w2863 = 2
                w2861 = FALSE ("1 6")
                n2172 = Select(t=0, s=w2868, f=1) -> (s? t:f=w2866:i32)
                n2173 = property on="均衡计算-电压高阀值1级" class="DigNum (严格)"("DisabledEnum"=w2866) -> ()  [unwired: 2 in, 2 out]
                n2174 = property on="均衡计算-电压高阀值2级" class="DigNum (严格)"("DisabledEnum"=w2866) -> ()  [unwired: 2 in, 2 out]
                n2175 = property on="均衡计算-电压低阀值1级" class="DigNum (严格)"("DisabledEnum"=w2866) -> ()  [unwired: 2 in, 2 out]
                n2176 = property on="均衡计算-电压低阀值2级" class="DigNum (严格)"("DisabledEnum"=w2866) -> ()  [unwired: 2 in, 2 out]
                n2177 = property on="均衡计算-最低电压阀值" class="DigNum (严格)"("DisabledEnum"=w2866) -> ()  [unwired: 2 in, 2 out]
                n2178 = property on="均衡停止-最低电压阀值" class="DigNum (严格)"("DisabledEnum"=w2866) -> ()  [unwired: 2 in, 2 out]
                n2179 = property on="均衡计算-电压极差阀值" class="DigNum (严格)"("DisabledEnum"=w2866) -> ()  [unwired: 2 in, 2 out]
                n2180 = property on="均衡参数" class="Clust (严格)"("DisabledEnum"=w2866) -> ()  [unwired: 2 in, 2 out]
                n2181 = property on="充电结束电压(90%)" class="DigNum (严格)"("DisabledEnum"=w2863) -> ()  [unwired: 2 in, 2 out]
                n2182 = property on="充电结束电压(91%)" class="DigNum (严格)"("DisabledEnum"=w2863) -> ()  [unwired: 2 in, 2 out]
                n2183 = property on="充电结束电压(92%)" class="DigNum (严格)"("DisabledEnum"=w2863) -> ()  [unwired: 2 in, 2 out]
                n2184 = property on="充电结束电压(93%)" class="DigNum (严格)"("DisabledEnum"=w2863) -> ()  [unwired: 2 in, 2 out]
                n2185 = property on="充电结束电压(94%)" class="DigNum (严格)"("DisabledEnum"=w2863) -> ()  [unwired: 2 in, 2 out]
                n2186 = property on="充电结束电压(95%)" class="DigNum (严格)"("DisabledEnum"=w2863) -> ()  [unwired: 2 in, 2 out]
                n2187 = property on="充电结束电压(96%)" class="DigNum (严格)"("DisabledEnum"=w2863) -> ()  [unwired: 2 in, 2 out]
                n2188 = property on="充电结束电压(97%)" class="DigNum (严格)"("DisabledEnum"=w2863) -> ()  [unwired: 2 in, 2 out]
                n2189 = property on="充电结束电压(98%)" class="DigNum (严格)"("DisabledEnum"=w2863) -> ()  [unwired: 2 in, 2 out]
                n2190 = property on="充电结束电压(99%)" class="DigNum (严格)"("DisabledEnum"=w2863) -> ()  [unwired: 2 in, 2 out]
                n2191 = property on="充电结束电压(100%)" class="DigNum (严格)"("DisabledEnum"=w2863) -> ()  [unwired: 2 in, 2 out]
                n2192 = disable-structure shown="启用" {
                  disable-tunnel: [w2872 w2874] -> w2865
                  disable-tunnel: [w2871 w2874] -> w2864
                  frame Enabled {
                    n2193 = global read "功能码全局.vi" "18"() -> (w2873:bool[])
                    n2194 = Index Array(array=w2873) -> (element #1=w2872:bool, element #2=w2871:bool)  [unwired: 8 in, 6 out]
                  }
                  frame Disabled {
                    w2874 = TRUE
                  }
                }
                n2195 = Not(x=w2861) -> (.not. x?=w2862:bool)
              }
              frame "充电结束电压" {
                w2878 = 2
                w2875 = FALSE ("1 6")
                n2196 = Select(t=0, s=w2882, f=1) -> (s? t:f=w2877:i32)
                n2197 = property on="均衡计算-电压高阀值1级" class="DigNum (严格)"("DisabledEnum"=w2878) -> ()  [unwired: 2 in, 2 out]
                n2198 = property on="均衡计算-电压高阀值2级" class="DigNum (严格)"("DisabledEnum"=w2878) -> ()  [unwired: 2 in, 2 out]
                n2199 = property on="均衡计算-电压低阀值1级" class="DigNum (严格)"("DisabledEnum"=w2878) -> ()  [unwired: 2 in, 2 out]
                n2200 = property on="均衡计算-电压低阀值2级" class="DigNum (严格)"("DisabledEnum"=w2878) -> ()  [unwired: 2 in, 2 out]
                n2201 = property on="均衡计算-最低电压阀值" class="DigNum (严格)"("DisabledEnum"=w2878) -> ()  [unwired: 2 in, 2 out]
                n2202 = property on="均衡停止-最低电压阀值" class="DigNum (严格)"("DisabledEnum"=w2878) -> ()  [unwired: 2 in, 2 out]
                n2203 = property on="均衡计算-电压极差阀值" class="DigNum (严格)"("DisabledEnum"=w2878) -> ()  [unwired: 2 in, 2 out]
                n2204 = property on="均衡参数" class="Clust (严格)"("DisabledEnum"=w2877) -> ()  [unwired: 2 in, 2 out]
                n2205 = property on="充电结束电压(90%)" class="DigNum (严格)"("DisabledEnum"=w2877) -> ()  [unwired: 2 in, 2 out]
                n2206 = property on="充电结束电压(91%)" class="DigNum (严格)"("DisabledEnum"=w2877) -> ()  [unwired: 2 in, 2 out]
                n2207 = property on="充电结束电压(92%)" class="DigNum (严格)"("DisabledEnum"=w2877) -> ()  [unwired: 2 in, 2 out]
                n2208 = property on="充电结束电压(93%)" class="DigNum (严格)"("DisabledEnum"=w2877) -> ()  [unwired: 2 in, 2 out]
                n2209 = property on="充电结束电压(94%)" class="DigNum (严格)"("DisabledEnum"=w2877) -> ()  [unwired: 2 in, 2 out]
                n2210 = property on="充电结束电压(95%)" class="DigNum (严格)"("DisabledEnum"=w2877) -> ()  [unwired: 2 in, 2 out]
                n2211 = property on="充电结束电压(96%)" class="DigNum (严格)"("DisabledEnum"=w2877) -> ()  [unwired: 2 in, 2 out]
                n2212 = property on="充电结束电压(97%)" class="DigNum (严格)"("DisabledEnum"=w2877) -> ()  [unwired: 2 in, 2 out]
                n2213 = property on="充电结束电压(98%)" class="DigNum (严格)"("DisabledEnum"=w2877) -> ()  [unwired: 2 in, 2 out]
                n2214 = property on="充电结束电压(99%)" class="DigNum (严格)"("DisabledEnum"=w2877) -> ()  [unwired: 2 in, 2 out]
                n2215 = property on="充电结束电压(100%)" class="DigNum (严格)"("DisabledEnum"=w2877) -> ()  [unwired: 2 in, 2 out]
                n2216 = disable-structure shown="启用" {
                  disable-tunnel: [w2886 w2888] -> w2880
                  disable-tunnel: [w2885 w2888] -> w2879
                  frame Enabled {
                    n2217 = global read "功能码全局.vi" "18"() -> (w2887:bool[])
                    n2218 = Index Array(array=w2887) -> (element #1=w2886:bool, element #2=w2885:bool)  [unwired: 8 in, 6 out]
                  }
                  frame Disabled {
                    w2888 = TRUE
                  }
                }
                n2219 = Not(x=w2875) -> (.not. x?=w2876:bool)
              }
              frame "假", Default {
                w2889 = FALSE ("1 6")
                n2220 = Not(x=w2889) -> (.not. x?=w2890:bool)
              }
            }
            n2221 = local write "等级 2"(w2480) -> ()
            n2222 = local write "1 6"(w2479) -> ()
            n2223 = local write "1 7"(w2478) -> ()
            n2224 = local write "1 8"(w2477) -> ()
            n2225 = local write "1 9"(w2476) -> ()
            n2226 = local write "1 10"(w2475) -> ()
            n2227 = local write "1 12"(w2469) -> ()
            n2228 = property on="单个读取" class="Bool (严格)"("Visible"=w2474) -> ()  [unwired: 2 in, 2 out]
            n2229 = property on="单个写入" class="Bool (严格)"("Visible"=w2473) -> ()  [unwired: 2 in, 2 out]
          }
          event "从板个数": Value Change {
            n2230 = event-data() -> ()  [unwired: 7 out]
            n2231 = local read "从板个数"() -> (w2892:dbl)
            n2232 = call "多从板对应参数-new.vi"("从板个数"=w2892) -> ("输出数组"=w2893:string[])  [unwired: 1 in]
            n2233 = control-ref of="项目信息"() -> (w2894:refnum<vi>)
